vi "I2C_WriteBitToSlave.vi"(8 "error in":errorcluster, 10 "Bit_Value":bool, 11 "HalfCycle(Ticks)":u32) -> (0 "error out":errorcluster)   [LabVIEW 2019]
doc: "Writes a Bit to the Slave Device.\n\n<b>Inputs:</b>\n--------------------\n<b>HalfCycle(Ticks)</b> this the number of FPGA clock cycles in half og the clock period. Therefore twice this number yields the clock period, in ticks.\n\n<b>PostAddressDelay(Ticks)</b> the delay in FPGA clock cycles before writing bytes on SDA.\n\nSee block diagram for more details on the implementation details.\n\nAuthor:\nPeter Fuller\nSenior Engineer\nPLF Consulting, LLC\n\nemail: peter@plfconsulting.com\nphone: 617.699.2201"
uses:
  <vilib>/eio/EIONode/EIONode.xnode
  Instance           1 27Saved   I2C_WriteBitToSlave .vi
  Instance           2 27Saved   I2C_WriteBitToSlave .vi
  <vilib>/eio/EIOMethodNode/EIOMethodNode.xnode
  <vilib>/rvi/eio/common/nirviEmuTemplateMethod_errors.vi
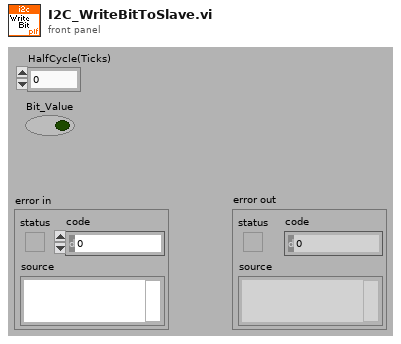
[diagram p1: front panel]
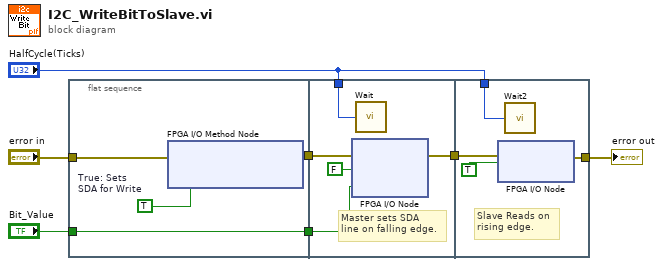
[diagram p0: block diagram]
diagram:
  n1 = flat-sequence {
    tunnel: "Bit_Value" -> [w11]
    tunnel: [w11] -> w6
    tunnel: "error in" -> [w9]
    tunnel: [w8] -> w4
    tunnel: w6 -> [w15]
    tunnel: w4 -> [w14]
    tunnel: [w13] -> w2
    tunnel: "HalfCycle(Ticks)" -> [w12]
    tunnel: w2 -> [w19]
    tunnel: "HalfCycle(Ticks)" -> [w17]
    tunnel: [w18] -> w3
    frame #0 {
      w10 = TRUE  # True: Sets  SDA for Write
      n2 = xnode "FPGA I/O Method Node"("error in"=w9, "Enable"=w10) -> ("error out"=w8:errorcluster)  [unwired: 1 in, 1 out]
    }
    frame #1 {
      # "Master sets SDA\nline on falling edge."
      n3 = xnode "FPGA I/O Node"("error in"=w14, "SCL"=FALSE ("Value"), "SDA"=w15) -> ("error out"=w13:errorcluster)  [unwired: 2 in, 2 out]
      n4 = call "Wait"("Count(Ticks)"=w12) -> ()  [unwired: 1 out]
    }
    frame #2 {
      # "Slave Reads on \nrising edge."
      n5 = xnode "FPGA I/O Node"("error in"=w19, "SCL"=TRUE ("Value")) -> ("error out"=w18:errorcluster)  [unwired: 1 in, 1 out]
      n6 = call "Wait2"("Count(Ticks)"=w17) -> ()  [unwired: 1 out]
    }
  }
  "error out" <- w3
